vi "JSON to LVObject.vi"(7 "LVClass Serializer":refnum<class "Generic Object Serializer.lvclass">, 8 "error in (no error)":errorcluster, 9 "Object Type":refnum<class>, 10 "Offset":i32, 11 "JSON":string) -> (0 "error out":errorcluster, 1 "Object":refnum<class>)   [LabVIEW 2017, in "Generic Object Serializer.lvclass"]
uses:
  Generic Object Serializer.lvclass
  C:/Program Files (x86)/National Instruments/LabVIEW 2017/vi.lib/JDP Science/JSONtext/LVClass Serializer/JSONtext LVClass Serializer.lvclass
  c49212c3-1964-49b6-8a35-88acbb3a007d.vi
  <vilib>/PNR/LabVIEW Composition/Composition/Get ClassName From Flattened Object.vi
  <vilib>/Utility/LVClass/Qualified Name Array To Single String.vi
  <vilib>/PNR/LabVIEW Composition/Composition/Composition.lvlib
  <vilib>/JDP Science/JSONtext/JSONtext.lvlib
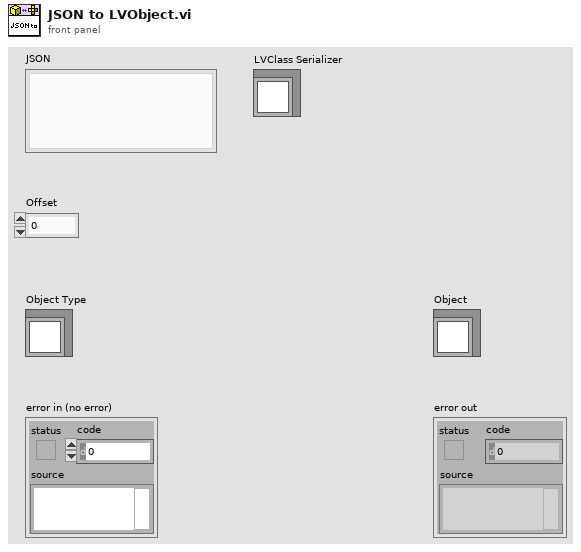
[diagram p1: front panel]
types:
  T1 = cluster{"Major":u16, "Minor":u16, "Fix":u16, "Build":u16}[]
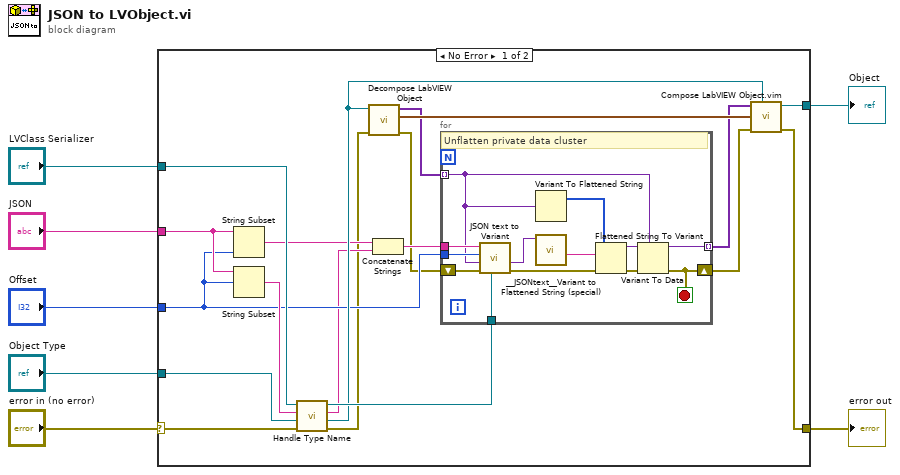
[diagram p0: block diagram]
diagram:
  n1 = case shown="No Error" "error in (no error)" {
    selector: "error in (no error)" -> [w17 w40]
    tunnel: "Object Type" -> [w21 _]
    tunnel: [w25 _] -> w6
    tunnel: "JSON" -> [w18 _]
    tunnel: "LVClass Serializer" -> [w23 _]
    tunnel: [w8 w40] -> w2
    tunnel: "Offset" -> [w13 _]
    frame No Error {
      n2 = String Subset(string=w18, length (rest)=w13) -> (substring=w16:string)  [unwired: 1 in]
      n3 = String Subset(string=w18, offset (0)=w13) -> (substring=w15:string)  [unwired: 1 in]
      n4 = call "Handle Type Name.vi"("error in (no error)"=w17, "Type"=w21, "JSON"=w15, "Flatten To JSON Object in"=w23) -> ("error out"=w11:errorcluster, "Type out"=w20:refnum<class>, "JSON out"=w12:string, "Flatten To JSON Object out"=w22:refnum<class "Generic Object Serializer.lvclass">)  [unwired: 4 in]
      n5 = call <vilib>:"Decompose LabVIEW Object.vi"("error in (no error)"=w11, "LabVIEW Object"=w20) -> ("error out"=w10:errorcluster, "Library Versions"=w26:T1, "Private Data Clusters"=w19:variant[])  [unwired: 6 in, 1 out]
      n6 = Concatenate Strings(w16, w12) -> (w14:string)
      n7 = for {
        tunnel: w14 -> [w37]
        tunnel: w19 -> [w32] mode=indexing
        tunnel: [w30] -> w24 mode=indexing
        tunnel: w22 -> [w38]
        tunnel: w13 -> [w39]
        shift-right: [w29] -> w9
        shift-left: w10 -> [w36]
        stop <- w29 stop-if-true
        # "Unflatten private data cluster"
        n8 = call <vilib>:"JSON text to Variant.vi"("LVClass Serializer"=w38, "error in (no error)"=w36, "Data Type"=w32, "Offset"=w39, "JSON"=w37) -> ("error out"=w31:errorcluster, "Variant out"=w28:variant)  [unwired: 5 in]
        n9 = Variant To Flattened String(Variant=w32) -> (1:w35:i16[])  [unwired: 1 out]
        n10 = call "__JSONtext__Variant to Flattened String (special).vi"("Variant"=w28) -> ("data"=w27:string)  [unwired: 9 in, 1 out]
        n11 = Flattened String To Variant(4:w31, 6:w27, 7:w35) -> (0:w33:errorcluster, 3:w34:variant)
        n12 = Variant To Data(error in=w33, type=w32, Variant=w34) -> (data=w30:variant, error out=w29:errorcluster)
      }
      n13 = call "Compose LabVIEW Object.vim"("Type"=w20, "error in (no error)"=w9, "Library Versions"=w26, "Private Data Clusters"=w24) -> ("error out"=w8:errorcluster, "LabVIEW Object"=w25:refnum<class>)  [unwired: 6 in]
    }
    frame Error {
    }
  }
  "error out" <- w2
  "Object" <- w6
